vi "Revision Query.vi"(8 "error in (no error)":errorcluster, 11 "VISA resource name":refnum<visa-resource-name>) -> (0 "error out":errorcluster, 1 "Instr Firmware Revision *":string, 2 "Instr Driver Revision":string, 3 "VISA resource name out":refnum<visa-resource-name>)   [LabVIEW 2020, in "Agilent 6XXX Series.lvlib"]
doc: "This VI queries the current instrument firmware revision and instrument driver revision. The Instrument Driver Revision: is \"Rev 1.0.1, 06/97, LV 4.1\", the Instrument Firmware Revision is Not Available\n\nHP 6030A\\31A\\32A\\33A\\35A\\38A,\nHP 6621A\\22A\\23A\\24A\\27A, & \nHP 6632A\\33A\\34A DC Power Supplies.\n\nCreated By: National Instruments\nRelease Date: October 1996\nOriginally Developed in LabVIEW Version: LV 4.0\n\nModification History: \n\n[JRO, 08 Apr 97]: Cosmetic changes, replaced the VISA session, dup VISA session, error in and error out controls because they were missing descriptions. Fixed the Menu palettes and changed the instrument driver revision number to \"Rev 1.0.1, 06/97, LV 4.1\" ."
uses:
  <instrlib>/Agilent 6XXX Series/Agilent 6XXX Series.lvlib
panel:
  # "*supported only on the HP663XA series"
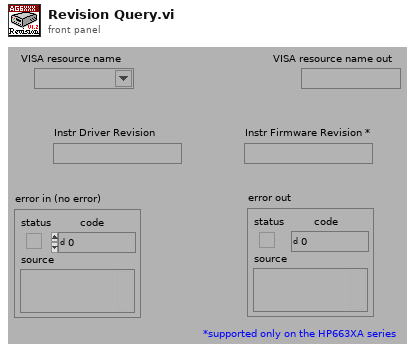
[diagram p1: front panel]
types:
  T1 = enum32{"invalid app kind", "Development System", "Run Time System", "Student Edition", "Embedded LabVIEW", "Evaluation", "Custom"}
  T2 = cluster{"Major":u16, "Minor":u16, "Fix":u16, "Build":u16}
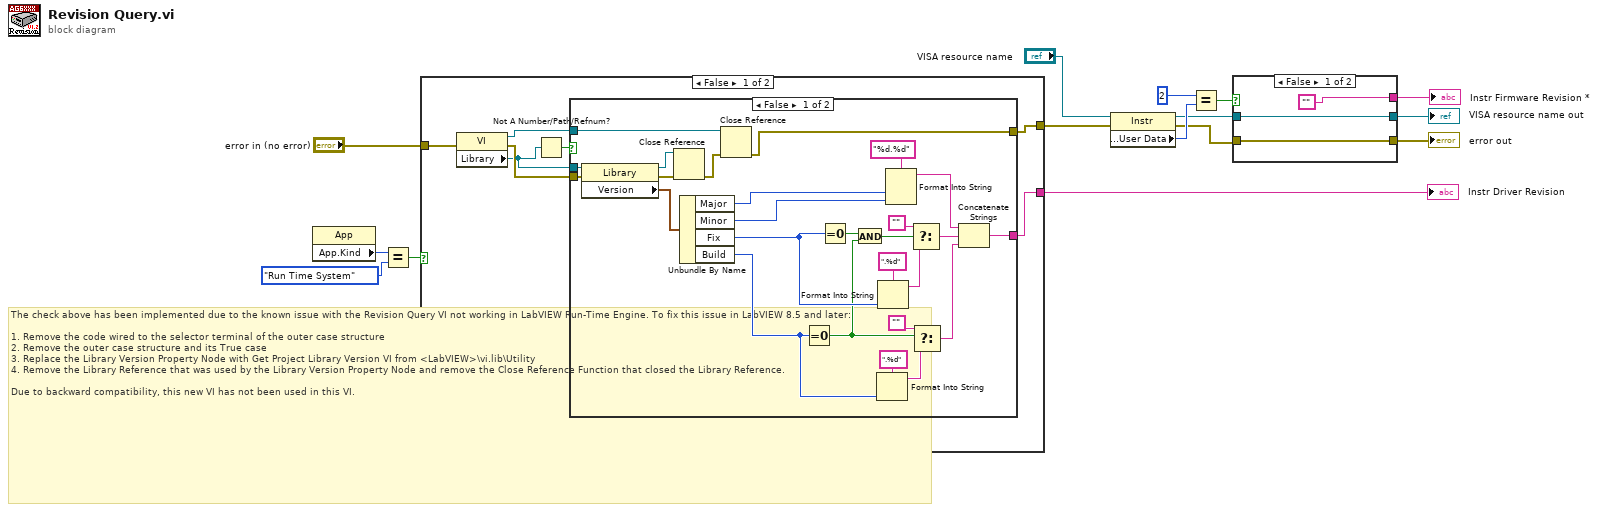
[diagram p0: block diagram]
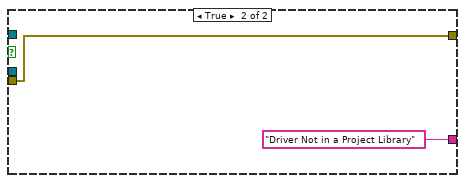
[diagram p2: hidden frame]
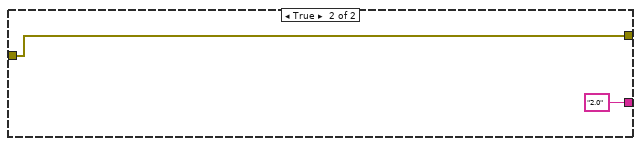
[diagram p3: hidden frame]
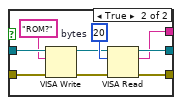
[diagram p4: hidden frame]
diagram:
  # "The check above has been implemented due to the known issue with the Revision Query VI not working in LabVIEW Run-Time Engine. To fix this issue in LabVIEW 8.5 and later:\n\n1. Remove the code wired to the selector terminal of the outer case structure\n2. Remove the outer case structure and its True case\n3. Replace the Library Version Property Node with Get Project Library Version VI from <LabVIEW>\\vi.lib\\Utility\n4. Remove the Library Reference that was used by the Library Version Property Node and remove the Close Reference Function that closed the Library Reference.\n\nDue to backward compatibility, this new VI has not been used in this VI."
  n1 = property class="App"() -> ("App.Kind"=w3:T1)  [unwired: 2 in, 2 out]
  n2 = Equal?(x=w3, y=T1."Run Time System") -> (x = y?=w1:bool)
  n3 = case shown="False" w1 {
    tunnel: "error in (no error)" -> [w22 w52]
    tunnel: [w17 "2.0"] -> w5
    tunnel: [w16 w52] -> w4
    frame False {
      n4 = property class="VI"(error in=w22) -> (reference out=w18:refnum<vi>, error out=w21:errorcluster, "Library"=w20:refnum<vi>)  [unwired: 1 in]
      n5 = Not A Number/Path/Refnum?(number/path/refnum=w20) -> (NaN/Path/Refnum?=w19:bool)
      n6 = case shown="False" w19 {
        tunnel: [w27 w49] -> w16
        tunnel: [w26 "Driver Not in a Project Library"] -> w17
        tunnel: w21 -> [w25 w49]
        tunnel: w20 -> [w24 _]
        tunnel: w18 -> [w23 _]
        frame False {
          n7 = property class="Library"(reference=w24, error in=w25) -> (reference out=w47:refnum<vi>, error out=w48:errorcluster, "Version"=w45:T2)
          n8 = Close Reference(reference=w47, error in (no error)=w48) -> (error out=w46:errorcluster)
          n9 = Unbundle By Name(w45) -> ("Major"=w34:u16, "Minor"=w33:u16, "Fix"=w31:u16, "Build"=w32:u16)
          n10 = Close Reference(reference=w23, error in (no error)=w46) -> (error out=w27:errorcluster)
          n11 = Equal To 0?(x=w32) -> (x = 0?=w29:bool)
          n12 = Equal To 0?(x=w31) -> (x = 0?=w30:bool)
          n13 = And(x=w30, y=w29) -> (x .and. y?=w28:bool)
          n14 = Format Into String(format string=".%d", w32) -> (resulting string=w38:string)  [unwired: 2 in, 1 out]
          n15 = Format Into String(format string=".%d", w31) -> (resulting string=w42:string)  [unwired: 2 in, 1 out]
          n16 = Format Into String(format string="%d.%d", w34, w33) -> (resulting string=w40:string)  [unwired: 2 in, 1 out]
          n17 = Select(t="", s=w28, f=w42) -> (s? t:f=w39:string)
          n18 = Select(t="", s=w29, f=w38) -> (s? t:f=w35:string)
          n19 = Concatenate Strings(w40, w39, w35) -> (w26:string)
        }
        frame True {
        }
      }
    }
    frame True {
    }
  }
  "Instr Driver Revision" <- w5
  n20 = property class="Instr"(reference="VISA resource name", error in=w4) -> (reference out=w8:refnum<visa-resource-name>, error out=w9:errorcluster, "General Settings:User Data"=w10:u32)
  n21 = Equal?(x=u32 2, y=w10) -> (x = y?=w14:bool)
  n22 = case shown="False" w14 {
    tunnel: w8 -> [w55 w60]
    tunnel: w9 -> [w54 w61]
    tunnel: [w55 w58] -> w13
    tunnel: [w54 w57] -> w11
    tunnel: ["" w56] -> w12
    frame False {
    }
    frame True {
      w64 = u32 20  # bytes
      n23 = VISA Write(VISA resource name=w60, write buffer="ROM?", error in (no error)=w61) -> (VISA resource name out=w63:refnum<visa-resource-name>, error out=w62:errorcluster)  [unwired: 1 out]
      n24 = VISA Read(VISA resource name=w63, byte count=w64, error in (no error)=w62) -> (VISA resource name out=w58:refnum<visa-resource-name>, read buffer=w56:string, error out=w57:errorcluster)  [unwired: 1 out]
    }
  }
  "error out" <- w11
  "Instr Firmware Revision *" <- w12
  "VISA resource name out" <- w13
